vi "Utility - Geokon8001 Read.vi"(8 "error in":errorcluster caption="错误输入（无错误）", 11 "VISA resource name":refnum<visa-resource-name>="COM2") -> (0 "error out":errorcluster caption="错误输出", 3 "Measurement Data":dbl[][](array[numeric]) caption="测量数据")   [LabVIEW 2015]
uses:
  <vilib>/Instr/_visa.llb/VISA Configure Serial Port (Instr).vi
panel:
  out "结果字符串":string
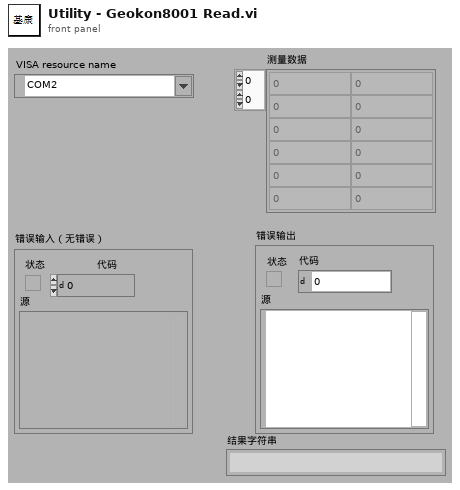
[diagram p1: front panel]
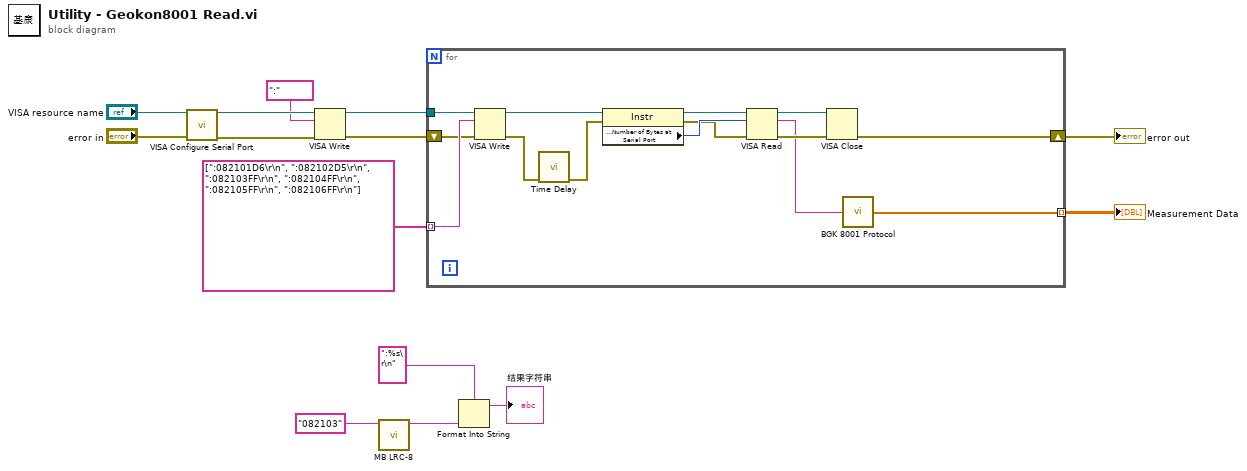
[diagram p0: block diagram]
diagram:
  n1 = call-poly "VISA Configure Serial Port"("VISA resource name"="VISA resource name", "error in (no error)"="error in") -> ("VISA resource name out"=w10:refnum<visa-resource-name>, "error out"=w8:errorcluster)  [unwired: 12 in]
  n2 = VISA Write(VISA resource name=w10, write buffer=":" ("写入缓冲区"), error in (no error)=w8) -> (VISA resource name out=w9:refnum<visa-resource-name>, error out=w7:errorcluster)  [unwired: 1 out]
  n3 = call "MB LRC-8.vi"("String"="082103" ("数据发送区")) -> ("string & LRC-8"=w3:string)  [unwired: 8 in, 2 out]
  n4 = for {
    tunnel: string[] [":082101D6\r\n", ":082102D5\r\n", ":082103FF\r\n", ":082104FF\r\n", ":082105FF\r\n", ":082106FF\r\n"] -> [w24] mode=indexing
    shift-right: [w19] -> w14
    shift-left: w7 -> [w18]
    tunnel: [w15] -> w13 mode=indexing
    tunnel: w9 -> [w17]
    n5 = VISA Write(VISA resource name=w17, write buffer=w24, error in (no error)=w18) -> (VISA resource name out=w20:refnum<visa-resource-name>, error out=w23:errorcluster)  [unwired: 1 out]
    n6 = call "Time Delay"("error in (no error)"=w23) -> ("error out"=w22:errorcluster)  [unwired: 10 in]
    n7 = property class="Instr"(reference=w20, error in=w22) -> (reference out=w21:refnum<visa-resource-name>, error out=w27:errorcluster, "Serial Settings:Number of Bytes at Serial Port"=w28:u32)
    n8 = VISA Read(VISA resource name=w21, byte count=w28, error in (no error)=w27) -> (VISA resource name out=w26:refnum<visa-resource-name>, read buffer=w16:string, error out=w25:errorcluster)  [unwired: 1 out]
    n9 = VISA Close(VISA resource name=w26, error in (no error)=w25) -> (error out=w19:errorcluster)
    n10 = call "BGK 8001 Protocol.vi"("字符串"=w16) -> ("数组"=w15:dbl[])
  }
  "error out" <- w14
  "Measurement Data" <- w13
  n11 = Format Into String(format string=":%s\r\n" ("格式字符串"), w3) -> (resulting string=→"结果字符串":string)  [unwired: 2 in, 1 out]
